vi "Simple Data Server.vi"() -> ()   [LabVIEW 2015]
doc: "This application shows how to use TCP communication to transfer streaming data from a RT target to a computer target. A TCP connection is opened between the targets, the data server on the RT target generates waveform data and transfers it via TCP to the data client on the computer target.\n\nInstructions:\n1. Open the Simple Data Client.vi.\n2. Run this VI first.\n3. Run the Simple Data Client.vi second.\n4. Adjust the Waveform and # of Points controls to see the plot on the front panel of the Simple Data Client.vi change.\n\nNote: This VI will time out after 60 seconds if no connection is detected."
uses:
  <vilib>/measure/NI_MABase.lvlib
panel:
  in  "Waveform":T1(ring)
  in  "Amplitude":dbl(slide)=5.0 scale=0.0..10.0
  in  "Frequency":dbl(slide)=5.0 scale=0.0..10.0
  in  "stop":bool
  in  "Port":u16=2055 min=1025 step=1
  # "This application shows how to use TCP communication to transfer \nstreaming data from a real-time target to your host PC.  A TCP \nconnection is opened between the targets, the data server on the \nRT target generates waveform data and transfers it via TCP to the \ndata client on your computer.\nInstructions:\n1. Open the Simple Data Client.vi.  \n2. Run this VI first (Simple Data Server.vi).\n3. Run the Simple Data Client.vi second.\n4. Adjust the Waveform Type, Frequency, and Amplitude controls \nto see the plot on the front panel of the Simple Data Client.vi update.\nNote:  This VI will time out after 60 seconds if no connection is detected."
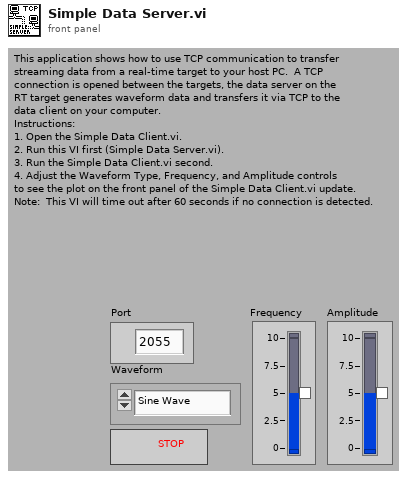
[diagram p1: front panel]
types:
  T1 = enum16{"Sine Wave", "Square Wave", "Sawtooth Wave", "White Noise"}
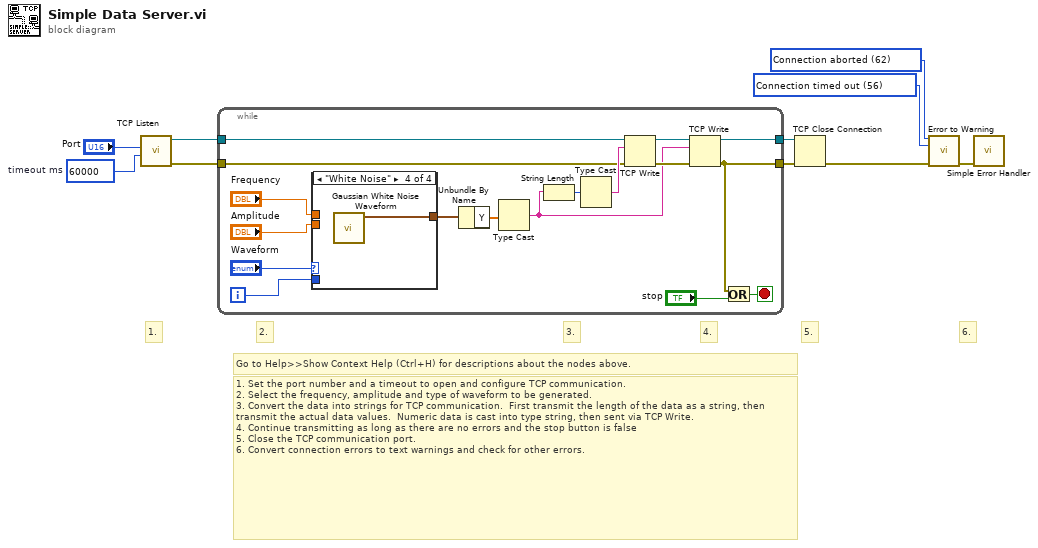
[diagram p0: block diagram]
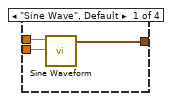
[diagram p2: hidden frame]
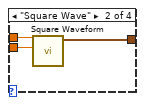
[diagram p3: hidden frame]
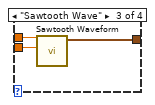
[diagram p4: hidden frame]
diagram:
  w2 = 60000  # timeout ms
  w7 = 56 items=["No Error", "Argument Error", "Memory Full", "Out of Zone", "End of File", "File Already Open", "Generic File IO Error", "File Not Found", "File Permission Error", "Disk Full", "Duplicate Path", "Too Many Files Open", "Not Enabled", "Resource File Not Found", "Cannot Add Resource", "Resource Not Found", "Image Not Found", "Image Memory Error", "Pen Does Not Exist", "Config Bad Type", "Config Token Not Found", "Config Parse Error", "Config Memory Error", "Bad External Code Format", "Bad External Code Offset", "External Code Not Present", "Null Window", "Destroy Window Mixup", "Null Menu", "Print Aborted", "Bad Print Record", "Print Driver Error", "Windows Error During Print", "Memory Error During Print", "Print Dialog Error", "Generic Print Error", "Invalid Device Refnum", "Device Not Found", "Device Parameter Error", "Device Unit Error", "Can't Open Device", "Device Call Aborted", "Generic Error", "Cancelled By User", "Object ID Too Low", "Object ID Too High", "Object Not In Heap", "Unknown Heap", "Bad DefProc ID", "DefProc Not In Table", "Message Out Of Range", "Null Method", "Unknown Message", "Manager Call Not Supported", "Bad address", "Connection In progress", "Connection timed out", "Connection is already in progress", "Network attribute not supported", "Network error", "Address in use", "System out of memory", "Connection aborted", "Connection refused", "Connection is not connected", "Connection is already connected", "Connection closed", "Initialize error (interapplication manager)", "Bad occurrence", "Wait on unbound occurrence handler", "Occurrence queue overflow", "Bad path", "Semaphore not signaled", "Unrecognized type (interapplication manager)"] ("2nd Error to Convert")
  w8 = 62 items=["No Error", "Argument Error", "Memory Full", "Out of Zone", "End of File", "File Already Open", "Generic File IO Error", "File Not Found", "File Permission Error", "Disk Full", "Duplicate Path", "Too Many Files Open", "Not Enabled", "Resource File Not Found", "Cannot Add Resource", "Resource Not Found", "Image Not Found", "Image Memory Error", "Pen Does Not Exist", "Config Bad Type", "Config Token Not Found", "Config Parse Error", "Config Memory Error", "Bad External Code Format", "Bad External Code Offset", "External Code Not Present", "Null Window", "Destroy Window Mixup", "Null Menu", "Print Aborted", "Bad Print Record", "Print Driver Error", "Windows Error During Print", "Memory Error During Print", "Print Dialog Error", "Generic Print Error", "Invalid Device Refnum", "Device Not Found", "Device Parameter Error", "Device Unit Error", "Can't Open Device", "Device Call Aborted", "Generic Error", "Cancelled By User", "Object ID Too Low", "Object ID Too High", "Object Not In Heap", "Unknown Heap", "Bad DefProc ID", "DefProc Not In Table", "Message Out Of Range", "Null Method", "Unknown Message", "Manager Call Not Supported", "Bad address", "Connection In progress", "Connection timed out", "Connection is already in progress", "Network attribute not supported", "Network error", "Address in use", "System out of memory", "Connection aborted", "Connection refused", "Connection is not connected", "Connection is already connected", "Connection closed", "Initialize error (interapplication manager)", "Bad occurrence", "Wait on unbound occurrence handler", "Occurrence queue overflow", "Bad path", "Semaphore not signaled", "Unrecognized type (interapplication manager)"] ("1st Error to Convert")
  # "Go to Help>>Show Context Help (Ctrl+H) for descriptions about the nodes above."
  # "6."
  # "5."
  # "4."
  # "3."
  # "2."
  # "1."
  # "1. Set the port number and a timeout to open and configure TCP communication.\n2. Select the frequency, amplitude and type of waveform to be generated.\n3. Convert the data into strings for TCP communication.  First transmit the length of the data as a string, then transmit the actual data values.  Numeric data is cast into type string, then sent via TCP Write.\n4. Continue transmitting as long as there are no errors and the stop button is false\n5. Close the TCP communication port.\n6. Convert connection errors to text warnings and check for other errors."
  n1 = call <vilib>:"TCP Listen.vi"("timeout ms (wait forever: -1)"=w2, "port"="Port") -> ("error out"=w3:errorcluster, "connection ID"=w5:refnum<k5>)  [unwired: 2 in, 6 out]
  n2 = while {
    tunnel: [w11] -> w4
    tunnel: [w27] -> w6
    tunnel: w5 -> [w26]
    tunnel: w3 -> [w15]
    i -> [w14]
    stop <- w20 stop-if-true
    n3 = case shown="\"White Noise\"" "Waveform" {
      tunnel: "Frequency" -> [w30 w33 w36 _]
      tunnel: "Amplitude" -> [w29 w32 w35 _]
      tunnel: w14 -> [_ _ _ _]
      tunnel: [w28 w31 w34 w37] -> w12
      frame "Sine Wave", Default {
        n4 = call <vilib>:"Sine Waveform.vi"("amplitude"=w29, "frequency"=w30) -> ("signal out"=w28:waveform(dbl))  [unwired: 5 in, 4 out]
      }
      frame "Square Wave" {
        n5 = call <vilib>:"Square Waveform.vi"("amplitude"=w32, "frequency"=w33) -> ("signal out"=w31:waveform(dbl))  [unwired: 6 in, 3 out]
      }
      frame "Sawtooth Wave" {
        n6 = call <vilib>:"Sawtooth Waveform.vi"("amplitude"=w35, "frequency"=w36) -> ("signal out"=w34:waveform(dbl))  [unwired: 5 in, 4 out]
      }
      frame "White Noise" {
        n7 = call <vilib>:"Gaussian White Noise Waveform.vi"() -> ("signal out"=w37:waveform(dbl))  [unwired: 5 in, 6 out]
      }
    }
    n8 = Unbundle By Name(w12) -> ("Y"=w13:dbl[])
    n9 = Type Cast(x=w13) -> (*(type *) &x=w21:string)  [unwired: 1 out]
    n10 = String Length(string=w21) -> (length=w23:i32)
    n11 = Type Cast(x=w23) -> (*(type *) &x=w22:string)  [unwired: 1 out]
    n12 = TCP Write(connection ID=w26, data in=w22, error in (no error)=w15) -> (connection ID out=w25:refnum<k5>, error out=w24:errorcluster)  [unwired: 2 out]
    n13 = TCP Write(connection ID=w25, data in=w21, error in (no error)=w24) -> (connection ID out=w27:refnum<k5>, error out=w11:errorcluster)  [unwired: 2 out]
    n14 = Or(x=w11, y="stop") -> (x .or. y?=w20:bool)
  }
  n15 = TCP Close Connection(connection ID=w6, error in (no error)=w4) -> (error out=w9:errorcluster)  [unwired: 2 out]
  n16 = call <vilib>:"Error to Warning.vi"("1st Error to Convert"=w8, "2nd Error to Convert"=w7, "error in"=w9) -> ("warning out"=w1:errorcluster)  [unwired: 3 in, 9 out]
  n17 = call <vilib>:"Simple Error Handler.vi"("error in (no error)"=w1) -> ()  [unwired: 1 in, 8 out]
